vi "ErrFrmRatio.vi"() -> ()   [LabVIEW 2017]
uses:
  globe.vi
panel:
  out "帧错误率(%)":dbl format="%#.2f"
  out "帧错误率波形图表":dbl(graph)
  out "接收帧数":dbl
  out "发送成功帧数":dbl
  out "总线错误帧数":dbl
  in  "刷新周期(ms)":u32=50 min=50 max=1000000
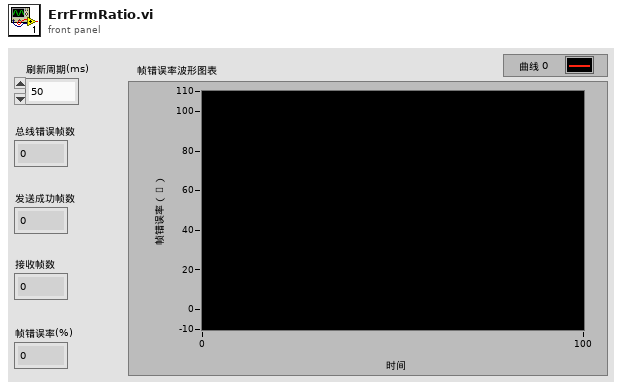
[diagram p1: front panel]
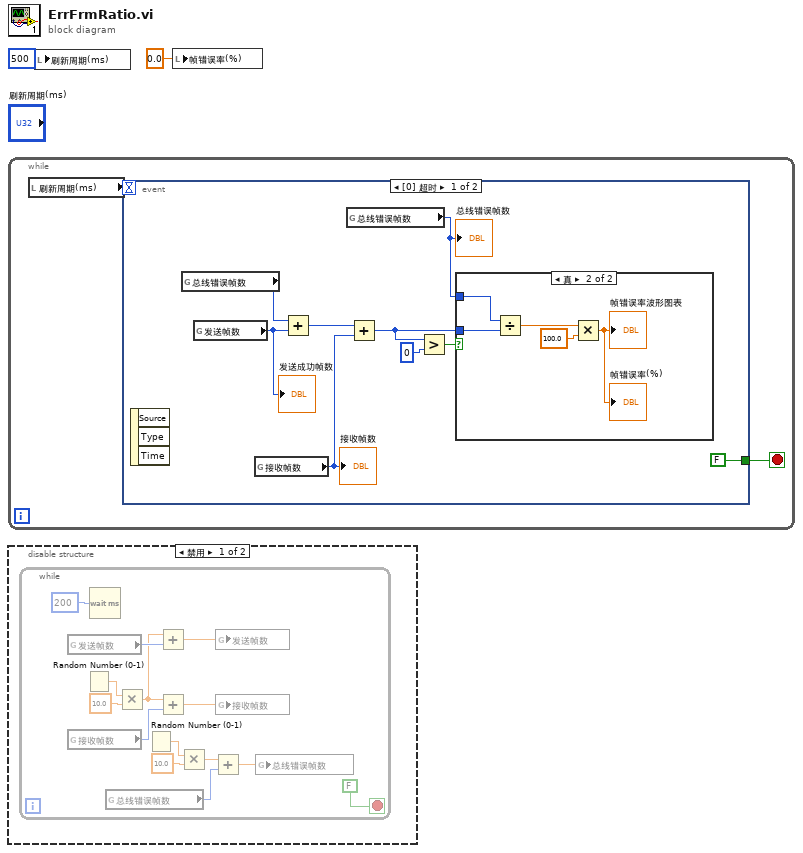
[diagram p0: block diagram]
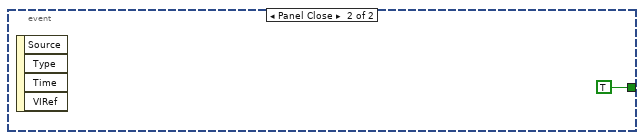
[diagram p4: hidden frame]
diagram:
  n1 = while {
    stop <- w4 stop-if-true
    n2 = local read "刷新周期(ms)"() -> (w3:u32)
    n3 = event shown="[0] 超时" {
      selector: _ -> [_ _]
      dyn-events: _ -> [_ _]
      timeout: w3 -> [_ _]
      tunnel: [FALSE TRUE ("停止")] -> w4
      event Timeout {
        n4 = event-data() -> ()  [unwired: 1 in, 3 out]
        n5 = global read "globe.vi" "总线错误帧数"() -> (w9:u32)
        n6 = global read "globe.vi" "发送帧数"() -> (w12:u32)
        "发送成功帧数" <- w12
        n7 = global read "globe.vi" "接收帧数"() -> (w10:u32)
        "接收帧数" <- w10
        n8 = Add(x=w9, y=w12) -> (x+y=w11:u32)
        n9 = global read "globe.vi" "总线错误帧数"() -> (w8:u32)
        "总线错误帧数" <- w8
        n10 = Add(x=w11, y=w10) -> (x+y=w6:u32)
        n11 = Greater?(x=w6, y=u32 0) -> (0:w7:bool)
        n12 = case shown="真" w7 {
          tunnel: w8 -> [_ w15]
          tunnel: w6 -> [_ w14]
          frame False {
          }
          frame True {
            n13 = Divide(x=w15, y=w14) -> (x/y=w18:dbl)
            n14 = Multiply(x=w18, y=100.0 ("x")) -> (x*y=→"帧错误率波形图表" →"帧错误率(%)":dbl)
          }
        }
      }
      event Panel Close {
        n15 = event-data() -> ()  [unwired: 1 in, 4 out]
      }
    }
  }
  n16 = disable-structure shown="禁用" {
    frame Disabled {
      n17 = while {
        stop <- FALSE stop-if-true
        n18 = global read "globe.vi" "发送帧数"() -> (w31:u32)
        n19 = global read "globe.vi" "接收帧数"() -> (w29:u32)
        n20 = Random Number (0-1)() -> (number: 0 to 1=w26:dbl)
        n21 = Wait (ms)(milliseconds to wait=u32 200 ("等待时间（毫秒）")) -> ()  [unwired: 1 out]
        n22 = global read "globe.vi" "总线错误帧数"() -> (w21:u32)
        n23 = Multiply(x=w26, y=10.0) -> (x*y=w25:dbl)
        n24 = Random Number (0-1)() -> (number: 0 to 1=w24:dbl)
        n25 = Add(x=w25, y=w31) -> (x+y=w30:dbl)
        n26 = Add(x=w25, y=w29) -> (x+y=w32:dbl)
        n27 = Multiply(x=w24, y=10.0) -> (x*y=w22:dbl)
        n28 = Add(x=w22, y=w21) -> (x+y=w20:dbl)
        n29 = global write "globe.vi" "发送帧数"(w30) -> ()
        n30 = global write "globe.vi" "接收帧数"(w32) -> ()
        n31 = global write "globe.vi" "总线错误帧数"(w20) -> ()
      }
    }
    frame Enabled {
    }
  }
  n32 = local write "刷新周期(ms)"(u32 500 ("刷新周期")) -> ()
  n33 = local write "帧错误率(%)"(0.0 ("帧错误率(%)")) -> ()
